vi "Write LV IMage.vi"(0 "Path":path, 1 "ImageDescription":string, 2 "Details":T6={"XResolution"=0.0, "YResolution"=0.0, "ResolutionUnit"=enum."Inch"}, 3 "Named Tags":T5(array[cluster]), 5 "image data":T7, 9 "operation (replace)":T1(ring)=enum."replace or create", 11 "error in (no error)":errorcluster, 12 "Compression":enum16{"None", "Deflate", "JPEG"}(ring), 13 "Settings":T2={"zlib compression level"=-1, "Max Strip bytes"=8192, "JPEG Quality (85)"=85}, 14 "Tags":T4(array[cluster])) -> (4 "path":path, 15 "error out":errorcluster)   [LabVIEW 2020, in "LV Tiff.lvlib" / "TIFF Writer.lvclass"]
uses:
  TIFF Writer.lvclass
  <vilib>/picture/picture.llb/imagedata.ctl
  _Helpers/Tiff Data Type.ctl
  _Helpers/Page Writer Settings.ctl
  _Helpers/Tiff Page Details.ctl
  LV Tiff.lvlib
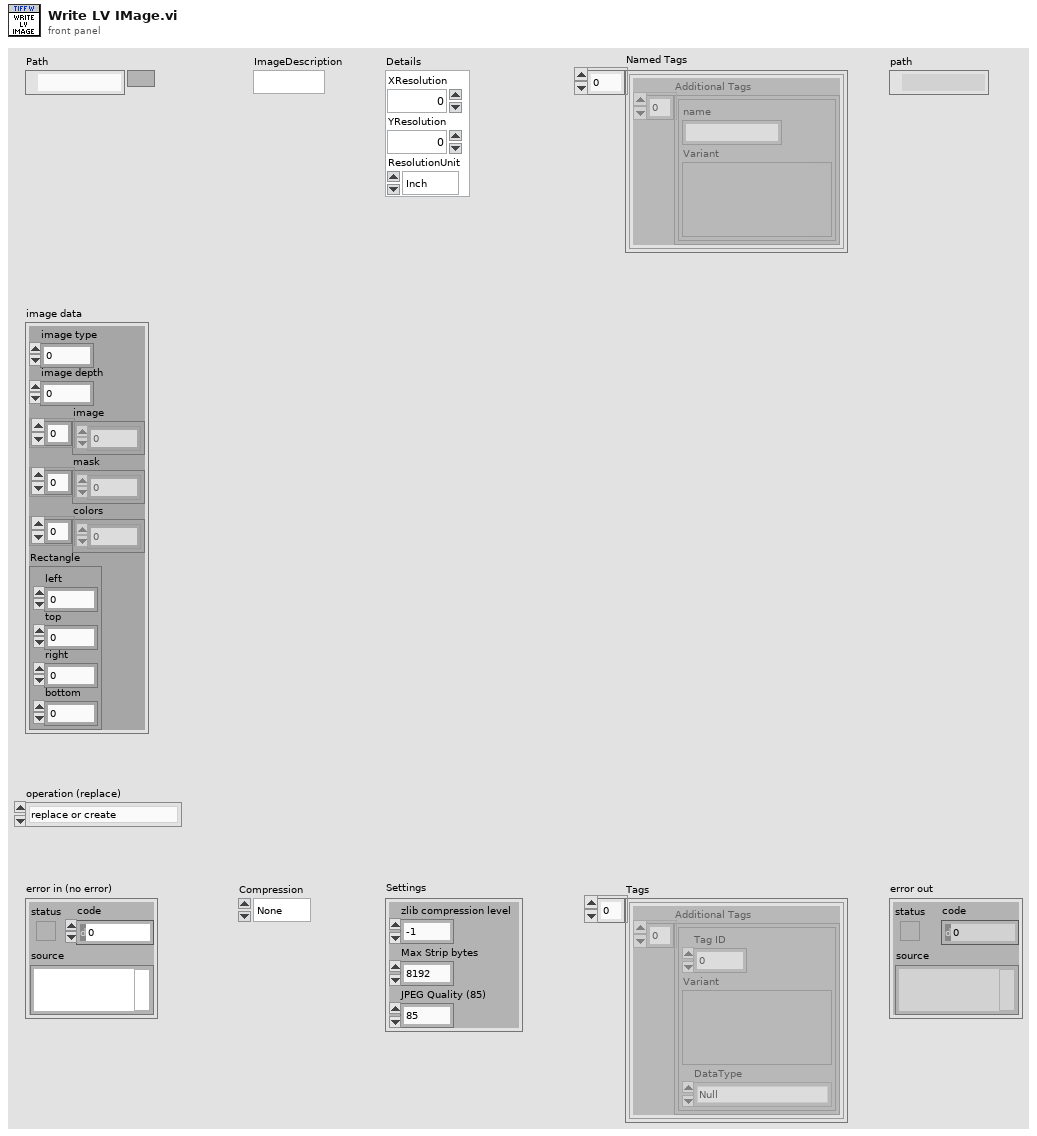
[diagram p1: front panel]
types:
  T1 = enum16{"open", "replace", "create", "open or create", "replace or create", "replace or create with confirmation"}
  T2 = typedef "LV Tiff.lvlib/Page Writer Settings.ctl" = cluster{"zlib compression level":i32, "Max Strip bytes":u32, "JPEG Quality (85)":i32}
  T3 = typedef "LV Tiff.lvlib/Tiff Data Type.ctl" = enum16{"Null", "BYTE", "ASCII", "SHORT", "LONG", "RATIONAL", "SBYTE", "UNDEFINE", "SSHORT", "SLONG", "SRATIONAL", "FLOAT", "DOUBLE"}
  T4 = cluster{"Additional Tags":cluster{"Tag ID":u32, "Variant":variant, "DataType":T3}[]}[]
  T5 = cluster{"Additional Tags":cluster{"name":string, "Variant":variant}[]}[]
  T6 = cluster{"XResolution":dbl, "YResolution":dbl, "ResolutionUnit":enum16{"None", "Inch", "Centimeter"}}
  T7 = typedef "imagedata.ctl" = cluster{"image type":i32, "image depth":i32, "image":u8[], "mask":u8[], "colors":u32[], "Rectangle":cluster{"left":i16, "top":i16, "right":i16, "bottom":i16}}
  T8 = typedef "LV Tiff.lvlib/Tiff Page Details.ctl" = cluster{"ImageDescription":string, "XResolution":dbl, "YResolution":dbl, "ResolutionUnit":enum16{"None", "Inch", "Centimeter"}, "PhotometricInterpretation":u16, "Compression":enum16{"None", "Deflate", "JPEG"}, "PageName":string, "DocumentName":string}
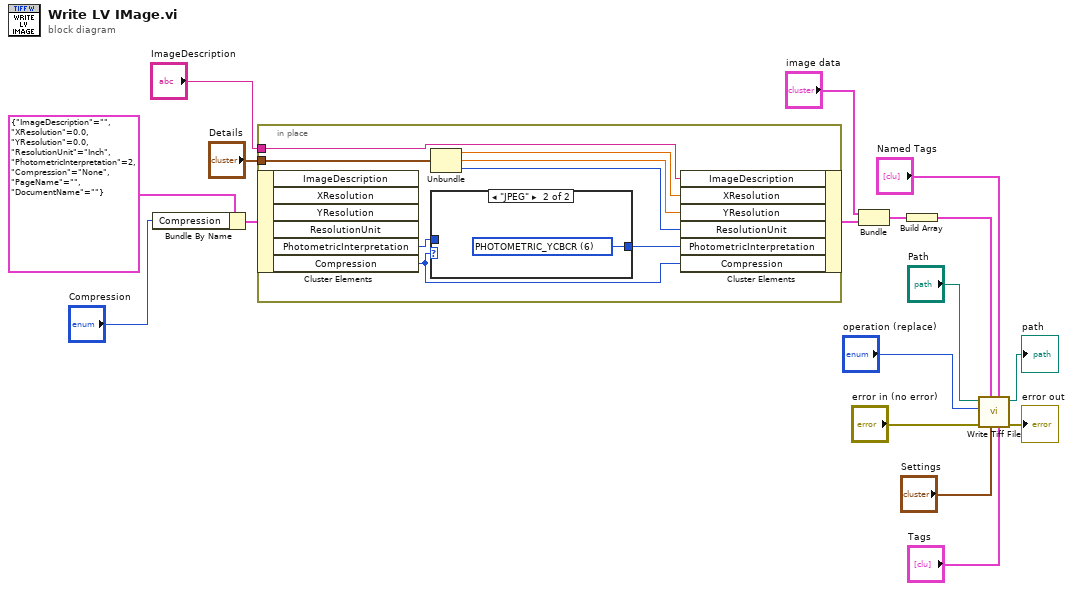
[diagram p0: block diagram]
diagram:
  n1 = Bundle By Name(cluster=T8 {"ImageDescription"="", "XResolution"=0.0, "YResolution"=0.0, "ResolutionUnit"=enum."Inch", "PhotometricInterpretation"=2, "Compression"=enum."None", "PageName"="", "DocumentName"=""} ("Details"), "Compression"="Compression") -> (w15:T8)
  n2 = in-place {
    in-place-border: "Details" -> [w22]
    in-place-border: "ImageDescription" -> [w18]
    n3 = in-place-cluster #1(w15) -> ("PhotometricInterpretation"=w23:u16, "Compression"=w25:enum16{"None", "Deflate", "JPEG"})  [unwired: 4 out]
    n4 = Unbundle(w22) -> ("XResolution"=w21:dbl, "YResolution"=w20:dbl, "ResolutionUnit"=w19:enum16{"None", "Inch", "Centimeter"})
    n5 = case shown="\"JPEG\"" w25 {
      tunnel: [w26 w27] -> w24
      tunnel: w23 -> [w26 _]
      frame Default {
      }
      frame "JPEG" {
        w27 = u16 6 items=["PHOTOMETRIC_MINISWHITE"=0, "PHOTOMETRIC_MINISBLACK"=1, "PHOTOMETRIC_RGB"=2, "PHOTOMETRIC_PALETTE"=3, "PHOTOMETRIC_MASK"=4, "PHOTOMETRIC_SEPARATED"=5, "PHOTOMETRIC_YCBCR"=6, "PHOTOMETRIC_CIELAB"=8, "PHOTOMETRIC_ICCLAB"=9, "PHOTOMETRIC_ITULAB"=10, "PHOTOMETRIC_LOGL"=32844, "PHOTOMETRIC_LOGLUV"=32845, "CFA"=32803, "LinearRaw"=34892, "DEPTH"=51177] ("PhotometricInterpretation")
      }
    }
    n6 = in-place-cluster #1("ImageDescription"=w18, "XResolution"=w21, "YResolution"=w20, "ResolutionUnit"=w19, "PhotometricInterpretation"=w24, "Compression"=w25) -> (w11:T8)
  }
  n7 = Bundle("image data"="image data", "Details"=w11) -> (w10:cluster{"image data":T7, "Details":T8})  [unwired: 1 in]
  n8 = Build Array(w10) -> (w9:cluster{"image data":T7, "Details":T8}[])
  n9 = call "Write Tiff File.vi"("Tags"="Tags", "Named Tags"="Named Tags", "Settings"="Settings", "Pages"=w9, "error in (no error)"="error in (no error)", "operation (replace)"="operation (replace)", "Path"="Path") -> ("error out"=→"error out":errorcluster, "path"=→"path":path)  [unwired: 3 in]
